vi "ke37xx Configure Display.vi"(0 "VISA Resource Name":refnum<visa-resource-name>, 5 "Clear Display (False)":bool, 9 "Message (Empty)":string, 11 "error in (no error)":errorcluster) -> (4 "VISA Resource Name Out":refnum<visa-resource-name>, 15 "error out":errorcluster)   [LabVIEW 2018, in "Keithley 3700 Series.lvlib"]
doc: "This VI controls the display on the front of the instrument."
uses:
  Keithley 3700 Series.lvlib
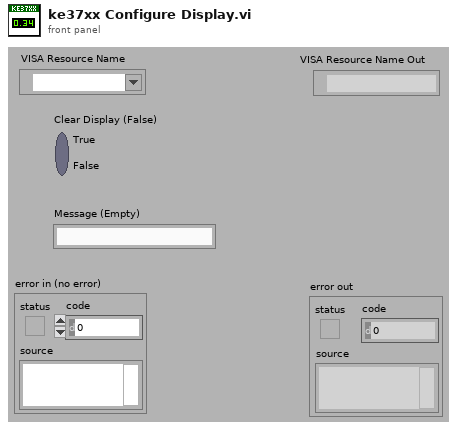
[diagram p1: front panel]
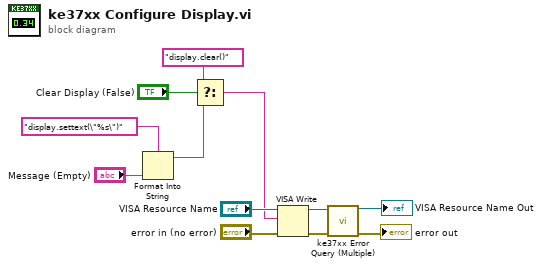
[diagram p0: block diagram]
diagram:
  n1 = Format Into String(format string="display.settext(\"%s\")", "Message (Empty)") -> (resulting string=w5:string)  [unwired: 2 in, 1 out]
  n2 = Select(t="display.clear()", s="Clear Display (False)", f=w5) -> (s? t:f=w9:string)
  n3 = VISA Write(VISA resource name="VISA Resource Name", write buffer=w9, error in (no error)="error in (no error)") -> (VISA resource name out=w4:refnum<visa-resource-name>, error out=w3:errorcluster)  [unwired: 1 out]
  n4 = call "ke37xx Error Query (Multiple).vi"("VISA resource name"=w4, "error in (no error)"=w3) -> ("VISA resource name out"=→"VISA Resource Name Out":refnum<visa-resource-name>, "error out"=→"error out":errorcluster)  [unwired: 12 out]
